vi "JGP5.vi"() -> ()   [LabVIEW 2019]
doc: "This Vi graphs original values of a 2d array and a squuare root values of the same 2d array\n\nJuan Gamez\nP3600\nCSUSB Physics"
panel:
  out "Data":dbl[][](graph)=[[0.0, 1.5, 3.0, 4.5, 6.0, 7.5, 9.0, 10.5, 12.0, 13.5, 15.0, 16.5, 18.0, 19.5, 21.0, 22.5, 24.0, 25.5, 27.0, 28.5, 30.0], [0.0, 1.224744871391589, 1.7320508075688772, 2.1213203435596424, 2.449489742783178, 2.7386127875258306, 3.0, 3.24037034920393, 3.4641016151377544, 3.6742346141747673, 3.872983346207417, 4.06201920231798, 4.242640687119285, 4.415880433163924, 4.58257569495584, 4.743416490252569, 4.898979485566356, 5.049752469181039, 5.196152422706632, 5.338539126015656, 5.477225575051661]]
  out "Spreadsheet column data":dbl[][](array[numeric])=[[0.0, 0.0], [1.5, 1.224744871391589], [3.0, 1.7320508075688772], [4.5, 2.1213203435596424], [6.0, 2.449489742783178], [7.5, 2.7386127875258306], [9.0, 3.0], [10.5, 3.24037034920393], [12.0, 3.4641016151377544], [13.5, 3.6742346141747673], [15.0, 3.872983346207417], [16.5, 4.06201920231798], [18.0, 4.242640687119285], [19.5, 4.415880433163924], [21.0, 4.58257569495584], [22.5, 4.743416490252569], [24.0, 4.898979485566356], [25.5, 5.049752469181039], [27.0, 5.196152422706632], [28.5, 5.338539126015656], [30.0, 5.477225575051661]]
  out "interval":dbl=1.5
  in  "N intervals":i32=20
  in  "end value":dbl=30.0
  in  "start value":dbl
  # "Juan Gamez\nP3600\nCsusb Physics"
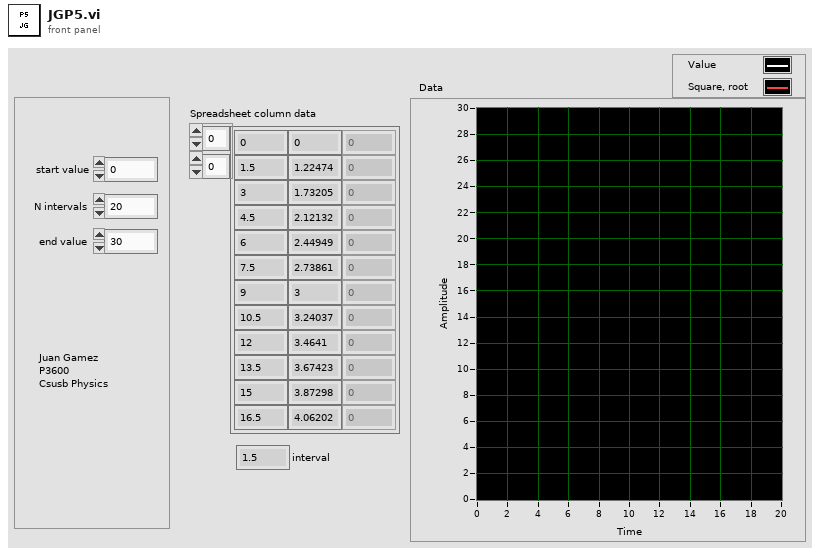
[diagram p1: front panel]
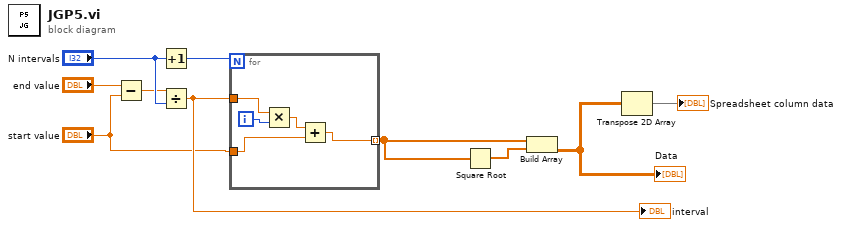
[diagram p0: block diagram]
diagram:
  n1 = Subtract(x="end value", y="start value") -> (x-y=w8:dbl)
  n2 = Increment(x="N intervals") -> (x+1=w7:i32)
  n3 = Divide(x=w8, y="N intervals") -> (x/y=w6:dbl)
  "interval" <- w6
  n4 = for {
    N: w7 -> [_]
    tunnel: w6 -> [w14]
    tunnel: "start value" -> [w12]
    tunnel: [w11] -> w3 mode=indexing
    i -> [w15]
    n5 = Multiply(x=w14, y=w15) -> (x*y=w13:dbl)
    n6 = Add(x=w13, y=w12) -> (x+y=w11:dbl)
  }
  n7 = Square Root(x=w3) -> (sqrt(x)=w4:dbl[])
  n8 = Build Array(w3, w4) -> (w2:dbl[][])
  "Data" <- w2
  n9 = Transpose 2D Array(2D array=w2) -> (transposed array=→"Spreadsheet column data":dbl[][])
